vi "OLD_RF_Attn_init.vi"(1 "Initialize Instrument":u64, 2 "Inst_param":T1) -> ()   [LabVIEW 2013]
uses:
  Attenuator_Vaunix-LDA_LabView_32Bit_Driver/Vaunix LDA/Vaunix LDA.lvlib
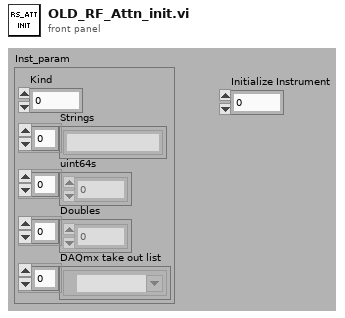
[diagram p1: front panel]
types:
  T1 = cluster{"Kind":u16, "Strings":string[], "uint64s":u64[], "Doubles":dbl[], "DAQmx take out list":refnum<k21>[]}
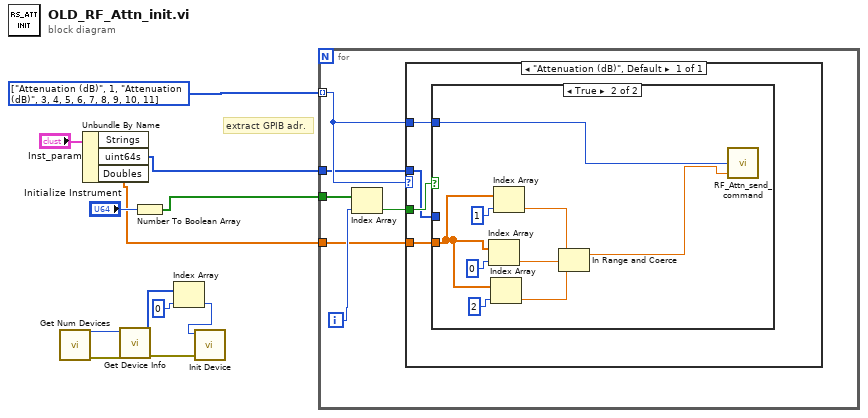
[diagram p0: block diagram]
diagram:
  w12 = enum16{"Attenuation (dB)"}[] [enum."Attenuation (dB)", 1, enum."Attenuation (dB)", 3, 4, 5, 6, 7, 8, 9, 10, 11] items=["Attenuation (dB)"]
  # "extract GPIB adr."
  n1 = call "Get Num Devices.vi"() -> ("error out"=w6:errorcluster, "Number of Devices"=w4:i32)  [unwired: 10 in]
  n2 = Unbundle By Name("Inst_param") -> ("uint64s"=w8:u64[], "Doubles"=w7:dbl[])  [unwired: 1 out]
  n3 = call "Get Device Info.vi"("error in (no error)"=w6, "Number of Devices"=w4) -> ("error out"=w5:errorcluster, "Active Devices"=w2:i32[])  [unwired: 7 in, 1 out]
  n4 = Number To Boolean Array(number="Initialize Instrument") -> (Boolean array=w9:bool[])
  n5 = Index Array(array=w2, index=0) -> (element=w1:i32)
  n6 = call "Init Device.vi"("error in (no error)"=w5, "Device ID in"=w1) -> ()  [unwired: 8 in, 2 out]
  n7 = for {
    tunnel: w12 -> [w16] mode=indexing
    tunnel: w9 -> [w18]
    tunnel: w8 -> [w14]
    tunnel: w7 -> [w13]
    i -> [w17]
    n8 = Index Array(array=w18, index=w17) -> (element=w15:bool)
    n9 = case shown="\"Attenuation (dB)\", Default" w16 {
      tunnel: w16 -> [w21]
      tunnel: w15 -> [w22]
      tunnel: w14 -> [w20]
      tunnel: w13 -> [w19]
      frame "Attenuation (dB)", Default {
        n10 = case shown="True" w22 {
          tunnel: w21 -> [_ w23]
          tunnel: w20 -> [_ _]
          tunnel: w19 -> [_ w26]
          frame False {
          }
          frame True {
            n11 = Index Array(array=w26, index=0) -> (element=w25:dbl)
            n12 = Index Array(array=w26, index=2) -> (element=w27:dbl)
            n13 = Index Array(array=w26, index=1) -> (element=w28:dbl)
            n14 = In Range and Coerce(upper limit=w28, x=w25, lower limit=w27) -> (coerced(x)=w24:dbl)  [unwired: 1 out]
            n15 = call "RF_Attn_send_command.vi"("Value"=w24, "Parameter"=w23) -> ()  [unwired: 2 in]
          }
        }
      }
    }
  }
